vi "Read Polling Iterations.vi"(8 "error in (no error)":errorcluster, 11 "Write Polling Iterations Msg in":refnum<class "Polling Iterations Msg.lvclass">) -> (0 "error out":errorcluster, 2 "Polling Iterations":u32, 3 "Write Polling Iterations Msg out":refnum<class "Polling Iterations Msg.lvclass">)   [LabVIEW 2016, in "CS++BaseActor.lvlib" / "Polling Iterations Msg.lvclass"]
uses:
  Polling Iterations Msg.lvclass
  Polling Iterations Msg.lvclass/Polling Iterations Msg.ctl
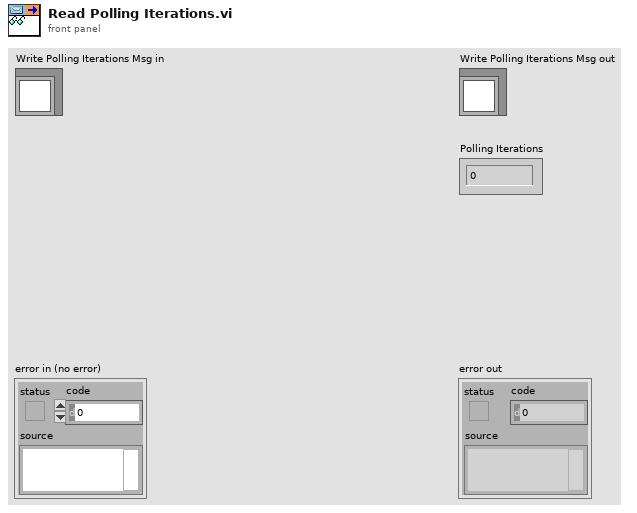
[diagram p1: front panel]
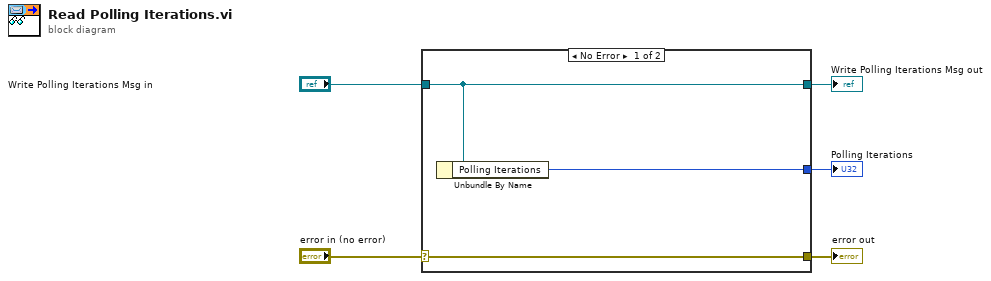
[diagram p0: block diagram]
diagram:
  n1 = case shown="No Error" "error in (no error)" {
    selector: "error in (no error)" -> [w8 w9]
    tunnel: [w8 w9] -> w4
    tunnel: [w7 w10] -> w2
    tunnel: "Write Polling Iterations Msg in" -> [w7 w10]
    tunnel: [w6 _] -> w1
    frame No Error {
      n2 = Unbundle By Name(w7) -> ("Polling Iterations"=w6:u32)
    }
    frame Error {
    }
  }
  "error out" <- w4
  "Write Polling Iterations Msg out" <- w2
  "Polling Iterations" <- w1
